vi "DP I-O Init Level.vi"(0 "StimGen":T1, 1 "DP Freqs":T2, 5 "DP stimulus params":T3={"Ear"=enum."Left", "f2 freqs (kHz)"="", "Start (dB)"=20.0, "Stop (dB)"=80.0, "Step (dB)"=10.0, "Mode"=enum."L1 = L2", "override recal"=FALSE, "Sampling Rate (Hz)"=0.0, "Frame (ms)"=0}, 11 "error in (no error)":errorcluster) -> (3 "StimGen Out":T1, 4 "Multipliers (2D)":dbl[][](array[numeric]), 6 "Gains (2D)":dbl[][](array[numeric]), 8 "Max SPL 1":dbl, 10 "Max SPL 2":dbl, 14 "Nominal f2 SPL":dbl[](array[numeric]), 15 "error out":errorcluster)   [LabVIEW 2020]
uses:
  Calibration VIs/CIE-2 Tone.vi
  epl-vi-lib/Utility VIs/Math VIs/LinSpace (start-stop-step).vi
  epl-vi-lib/PXI DAQ VIs/DAQ Engine VIs/AO Gain and Multiplier VIs/PXI Multipliers to AO Gains (1D).vi
  Utility VIs/Math VIs/dB to Linear (1D).vi
  Typedefs/DP Stimulus Params.ctl
  Typedefs/DP-StimGen.ctl
  Typedefs/DP-Freqs.ctl
panel:
  out "Nominal f1 SPL":dbl[](array[numeric])
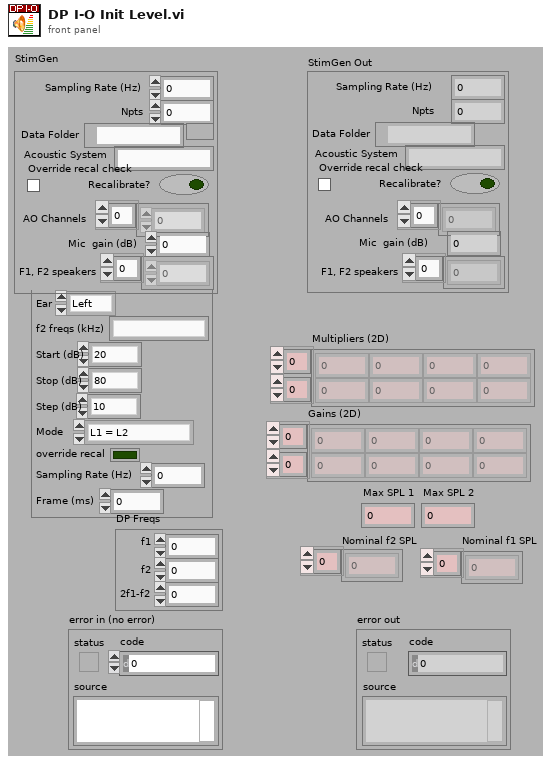
[diagram p1: front panel]
types:
  T1 = typedef "DP-StimGen.ctl" = cluster{"Sampling Rate (Hz)":dbl, "Npts":i32, "Data Folder":path, "Acoustic System":string, "Recalibrate?":bool, "AO Channels":i32[], "Mic  gain (dB)":dbl, "F1, F2 speakers":i32[], "Override recal check":bool}
  T2 = typedef "DP-Freqs.ctl" = cluster{"f1":dbl, "f2":dbl, "2f1-f2":dbl}
  T3 = typedef "DP Stimulus Params.ctl" = cluster{"Ear":enum16{"Right", "Left"}, "f2 freqs (kHz)":string, "Start (dB)":dbl, "Stop (dB)":dbl, "Step (dB)":dbl, "Mode":enum16{"L1 = L2", "L1 = L2 + 10 dB"}, "override recal":bool, "Sampling Rate (Hz)":dbl, "Frame (ms)":i32}
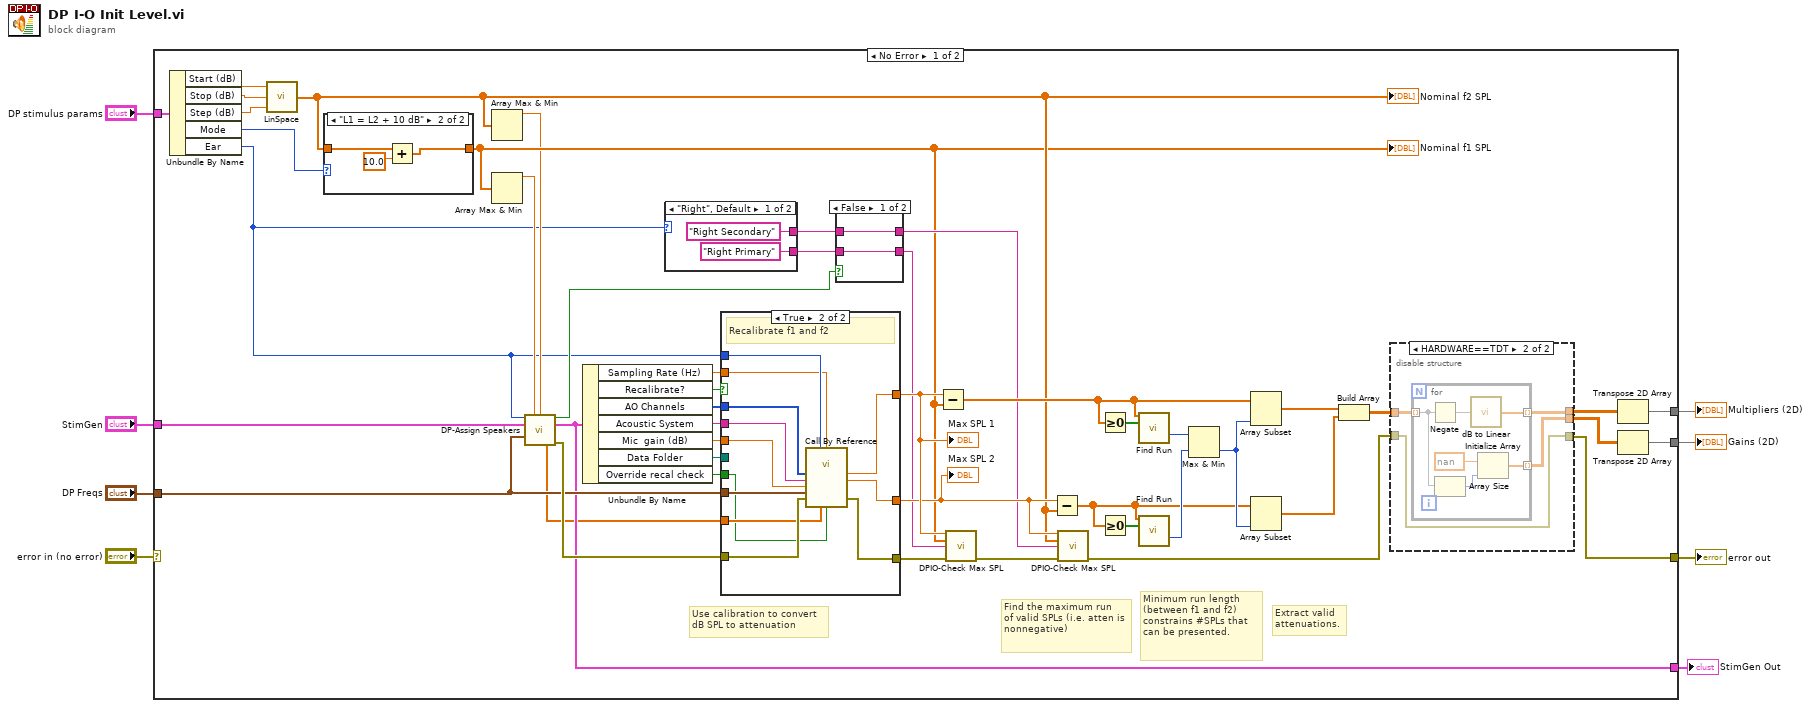
[diagram p0: block diagram]
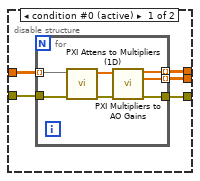
[diagram p2: hidden frame]
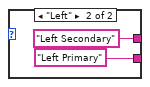
[diagram p4: hidden frame]
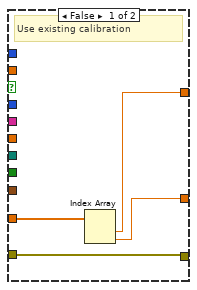
[diagram p5: hidden frame]
diagram:
  n1 = case shown="No Error" "error in (no error)" {
    selector: "error in (no error)" -> [_ w106]
    tunnel: "DP stimulus params" -> [w25 _]
    tunnel: [w46 w106] -> w7
    tunnel: [w41 _] -> w5
    tunnel: [w40 _] -> w4
    tunnel: "DP Freqs" -> [w24 _]
    tunnel: "StimGen" -> [w27 _]
    tunnel: [w17 _] -> w1
    frame No Error {
      # "Extract valid attenuations."
      # "Minimum run length (between f1 and f2) constrains #SPLs that can be presented."
      # "Find the maximum run\nof valid SPLs (i.e. atten is nonnegative)"
      # "Use calibration to convert\ndB SPL to attenuation"
      n2 = Unbundle By Name(w25) -> ("Start (dB)"=w55:dbl, "Stop (dB)"=w54:dbl, "Step (dB)"=w53:dbl, "Mode"=w52:enum16{"L1 = L2", "L1 = L2 + 10 dB"}, "Ear"=w12:enum16{"Right", "Left"})
      n3 = call-poly "LinSpace.vi"("Step"=w53, "Stop"=w54, "Start"=w55) -> ("Array"=w16:dbl[])  [unwired: 1 in, 1 out]
      "Nominal f2 SPL" <- w16
      n4 = case shown="\"L1 = L2 + 10 dB\"" w52 {
        tunnel: w16 -> [w102 w105]
        tunnel: [w102 w103] -> w15
        frame "L1 = L2", Default {
        }
        frame "L1 = L2 + 10 dB" {
          n5 = Add(x=w105, y=10.0 ("Numeric")) -> (x+y=w103:dbl[])
        }
      }
      "Nominal f1 SPL" <- w15
      n6 = Array Max & Min(array=w16) -> (max value=w14:dbl)  [unwired: 3 out]
      n7 = Array Max & Min(array=w15) -> (max value=w13:dbl)  [unwired: 3 out]
      n8 = call "DP-Assign Speakers.vi"("Ear"=w12, "F1 Max Req"=w13, "F2 Max  Req"=w14, "StimGen In"=w27, "DP Freqs"=w24) -> ("Flipped?"=w23:bool, "StimGen Out"=w17:T1, "Nominal Max SPL"=w11:dbl[], "error out"=w26:errorcluster)  [unwired: 7 in]
      n9 = Unbundle By Name(w17) -> ("Sampling Rate (Hz)"=w9:dbl, "Recalibrate?"=w35:bool, "AO Channels"=w18:i32[], "Acoustic System"=w33:string, "Mic  gain (dB)"=w32:dbl, "Data Folder"=w34:path, "Override recal check"=w10:bool)
      n10 = case shown="\"Right\", Default" w12 {
        tunnel: ["Right Primary" "Left Primary"] -> w22
        tunnel: ["Right Secondary" "Left Secondary"] -> w21
        frame "Right", Default {
        }
        frame "Left" {
        }
      }
      n11 = case shown="True" w35 {
        tunnel: w26 -> [w89 w101]
        tunnel: [w89 w99] -> w48
        tunnel: [w87 w100] -> w30
        tunnel: w34 -> [_ _]
        tunnel: w12 -> [_ w97]
        tunnel: [w86 w98] -> w28
        tunnel: w33 -> [_ w94]
        tunnel: w32 -> [_ w95]
        tunnel: w24 -> [_ w96]
        tunnel: w18 -> [_ w93]
        tunnel: w11 -> [w88 w92]
        tunnel: w10 -> [_ w91]
        tunnel: w9 -> [_ w90]
        frame False {
          # "Use existing calibration"
          n12 = Index Array(array=w88) -> (element #1=w87:dbl, element #2=w86:dbl)  [unwired: 2 in]
        }
        frame True {
          # "Recalibrate f1 and f2"
          n13 = call-by-ref "?"("AO Channels"=w93, "Ear"=w97, "Sampling Rate (Hz)"=w90, "Acoustic System"=w94, "Probe mic gain (dB)"=w95, "DP Freqs"=w96, "error in (no error)"=w101, "Nominal Max SPLs"=w92, "Override recal check?"=w91) -> ("Max SPL1"=w100:dbl, "Max SPL2"=w98:dbl, "error out"=w99:errorcluster)  [unwired: 6 in, 2 out]
        }
      }
      "Max SPL 1" <- w30
      "Max SPL 2" <- w28
      n14 = case shown="False" w23 {
        tunnel: w22 -> [w78 w80]
        tunnel: w21 -> [w79 w81]
        tunnel: [w79 w80] -> w20
        tunnel: [w78 w81] -> w19
        frame False {
        }
        frame True {
        }
      }
      n15 = Subtract(x=w30, y=w15) -> (x-y=w39:dbl[])
      n16 = call "DPIO-Check Max SPL.vi"("Max SPL"=w30, "SPL Array"=w15, "Channel"=w19, "error in (no error)"=w48) -> ("error out"=w31:errorcluster)  [unwired: 11 in]
      n17 = Subtract(x=w28, y=w16) -> (x-y=w38:dbl[])
      n18 = call "DPIO-Check Max SPL.vi"("Max SPL"=w28, "SPL Array"=w16, "Channel"=w20, "error in (no error)"=w31) -> ("error out"=w29:errorcluster)  [unwired: 11 in]
      n19 = Greater Or Equal To 0?(x=w39) -> (x >= 0?=w51:bool[])
      n20 = Greater Or Equal To 0?(x=w38) -> (x >= 0?=w36:bool[])
      n21 = call "Find Run.vi"("Array"=w39, "Condition"=w51) -> ("Run length"=w50:i32)  [unwired: 10 in, 3 out]
      n22 = call "Find Run.vi"("Array"=w38, "Condition"=w36) -> ("Run length"=w49:i32)  [unwired: 10 in, 3 out]
      n23 = Max & Min(x=w50, y=w49) -> (min(x,y)=w47:i32)  [unwired: 1 out]
      n24 = Array Subset(array=w39, length=w47) -> (w43:dbl[])  [unwired: 1 in]
      n25 = Array Subset(array=w38, length=w47) -> (w37:dbl[])  [unwired: 1 in]
      n26 = Build Array(w43, w37) -> (w42:dbl[][])
      n27 = disable-structure shown="HARDWARE==TDT" {
        disable-tunnel: [w60 w68] -> w46
        disable-tunnel: [w59 w70] -> w45
        disable-tunnel: [w58 w69] -> w44
        disable-tunnel: w42 -> [w57 w71]
        disable-tunnel: w29 -> [w56 w68]
        frame condition #0 (active) {
          n28 = for {
            tunnel: w56 -> [w67]
            tunnel: [w66] -> w60
            tunnel: [w65] -> w59 mode=indexing
            tunnel: [w64] -> w58 mode=indexing
            tunnel: w57 -> [w61] mode=indexing
            n29 = call "PXI Attens to Multipliers (1D).vi"("error in (no error)"=w67, "Array of Attens"=w61) -> ("error out"=w62:errorcluster, "Multiplier setting"=w63:dbl[])  [unwired: 8 in]
            n30 = call-poly "PXI Multipliers to AO Gains.vi"("Multipliers in"=w63, "error in (no error)"=w62) -> ("Multipliers out"=w65:dbl[], "Gains"=w64:dbl[], "error out"=w66:errorcluster)  [unwired: 11 in]
          }
        }
        frame condition #1 {
          n31 = for {
            tunnel: w71 -> [w73] mode=indexing
            tunnel: [w77] -> w70 mode=indexing
            tunnel: [w75] -> w69 mode=indexing
            n32 = Negate(x=w73) -> (-x=w72:dbl[])
            n33 = Array Size(array=w73) -> (size(s)=w74:i32)
            n34 = call-poly "dB to Linear.vi"("dB"=w72) -> ("linear"=w77:dbl[])
            n35 = Initialize Array(nan, w74) -> (w75:dbl[])
          }
        }
      }
      n36 = Transpose 2D Array(2D array=w45) -> (transposed array=w41:dbl[][])
      n37 = Transpose 2D Array(2D array=w44) -> (transposed array=w40:dbl[][])
    }
    frame Error {
    }
  }
  "error out" <- w7
  "Multipliers (2D)" <- w5
  "Gains (2D)" <- w4
  "StimGen Out" <- w1
